vi "GetServerNamesAndContents.vi"(0 "Desired Server":i32) -> (1 "Label":string, 2 "Queue Contents":string[](array[string]), 3 "Nice Names":string[][](array[string]), 4 "Symbols":i32[](array[numeric]))   [LabVIEW 2012]
uses:
  <userlib>/ROS for LabVIEW Software/ROS/Code/_ROSDefinition.vi
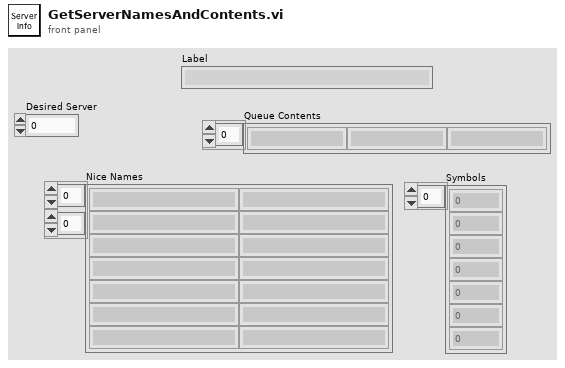
[diagram p1: front panel]
types:
  T1 = typedef "_ROSControl.ctl" = cluster{"topic port":u16, "Node":string, "topic":string, "type":string, "node port":u16, "error ":errorcluster, "Direction":T2, "Update (ms)":u16, "FIFO size":u16}
  T2 = typedef "_ROSDirection.ctl" = enum16{"Node", "Publisher", "Subscriber", "ServiceClient", "ServiceProvider"}
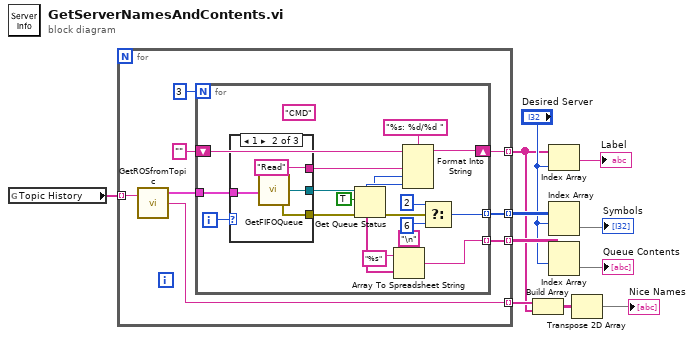
[diagram p0: block diagram]
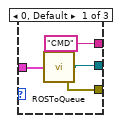
[diagram p2: hidden frame]
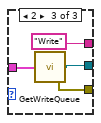
[diagram p3: hidden frame]
diagram:
  n1 = global read "_ROSDefinition.vi" "Topic History"() -> (w11:string[])
  n2 = for {
    tunnel: w11 -> [w19] mode=indexing
    tunnel: [w18] -> w4 mode=indexing
    tunnel: [w14] -> w7 mode=indexing
    tunnel: [w13] -> w9 mode=indexing
    tunnel: [w12] -> w3 mode=indexing
    n3 = call <userlib>:"GetROSfromTopic.vi"("Topic"=w19) -> ("ROS"=w17:T1, "Nice Name"=w18:string)  [unwired: 1 in, 1 out]
    n4 = for {
      N: 3 -> [_]
      tunnel: w17 -> [w29]
      shift-right: [w30] -> w12
      shift-left: "" -> [w31]
      tunnel: [w20] -> w14 mode=indexing
      tunnel: [w24] -> w13 mode=indexing
      i -> [w38]
      (unwired) "CMD"
      n5 = case shown="1" w38 {
        tunnel: w29 -> [w42 w45 w50]
        tunnel: [w41 w46 w49] -> w28
        tunnel: [w40 w44 w48] -> w27
        tunnel: ["CMD" "Read" "Write"] -> w25
        frame 0, Default {
          n6 = call <userlib>:"ROSToQueue.vi"("ROS"=w42) -> ("error out"=w40:errorcluster, "queue"=w41:refnum<queue>)  [unwired: 3 in]
        }
        frame 1 {
          n7 = call <userlib>:"GetFIFOQueue.vi"("ROS"=w45) -> ("error out"=w44:errorcluster, "queue out"=w46:refnum<queue>)  [unwired: 3 in]
        }
        frame 2 {
          n8 = call <userlib>:"GetWriteQueue.vi"("ROS"=w50) -> ("error out"=w48:errorcluster, "queue out"=w49:refnum<queue>)  [unwired: 3 in]
        }
      }
      n9 = Get Queue Status(queue=w28, return elements? (F)=TRUE, error in (no error)=w27) -> (max queue size=w33:i32, error out=w35:errorcluster, # elements in queue=w26:i32, elements=w21:string[])  [unwired: 4 out]
      n10 = Array To Spreadsheet String(delimiter (Tab)="\n", array=w21, 3:"%s" ("format string")) -> (spreadsheet string=w20:string)
      n11 = Format Into String(format string="%s: %d/%d ", initial string=w31, w25, w26, w33) -> (resulting string=w30:string)  [unwired: 1 in, 1 out]
      n12 = Select(t=2, s=w35, f=6) -> (s? t:f=w24:i32)
    }
  }
  n13 = Build Array(w4, w3) -> (w2:string[][])
  n14 = Index Array(array=w3, index="Desired Server") -> (element=→"Label":string)
  n15 = Index Array(array=w9, index (row)="Desired Server") -> (element=→"Symbols":i32[])  [unwired: 1 in]
  n16 = Index Array(array=w7, index (row)="Desired Server") -> (element=→"Queue Contents":string[])  [unwired: 1 in]
  n17 = Transpose 2D Array(2D array=w2) -> (transposed array=→"Nice Names":string[][])
